vi "HXG2_Timing Module Pump.vi"(7 "Timer Command":T1=enum."Start", 8 "error in (no error)":errorcluster) -> (0 "error out":errorcluster, 1 "Elapsed Time":dbl, 2 "Done?":bool)   [LabVIEW 2012]
doc: "This VI is a functional global variable that keeps track the amount of time elapsed since a Start command was sent to the VI."
uses:
  HXG2_BlowerPumpl.ctl
panel:
  # "Input"
  # "Output"
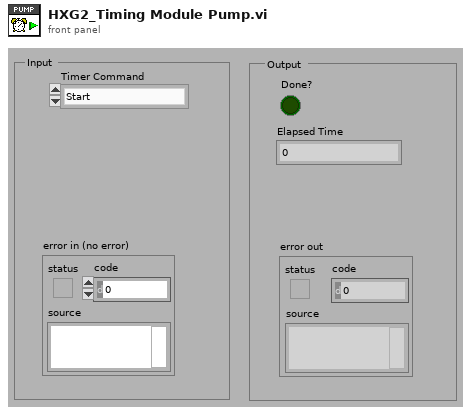
[diagram p1: front panel]
types:
  T1 = typedef "HXG2_BlowerPumpl.ctl" = enum16{"Stop", "Start", "Check Time"}
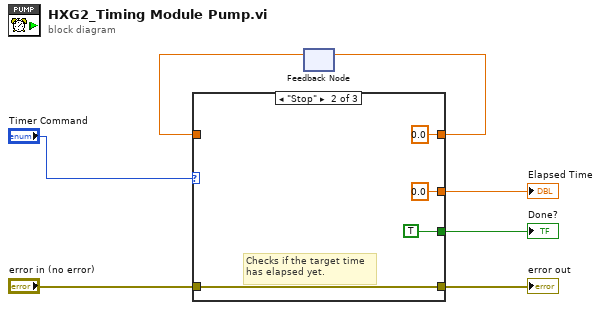
[diagram p0: block diagram]
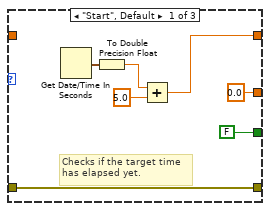
[diagram p2: hidden frame]
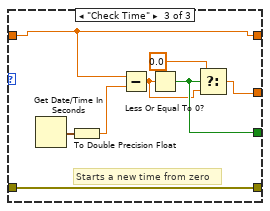
[diagram p3: hidden frame]
diagram:
  n1 = feedback #1() -> (w3:dbl)  [unwired: 1 in]
  n2 = case shown="\"Stop\"" "Timer Command" {
    tunnel: [w10 0.0 w19] -> w4
    tunnel: w3 -> [_ _ w19]
    tunnel: [0.0 ("t") 0.0 ("t") w23] -> w7
    tunnel: [FALSE TRUE w22] -> w6
    tunnel: "error in (no error)" -> [w12 w18 w26]
    tunnel: [w12 w18 w26] -> w1
    frame "Start", Default {
      # "Checks if the target time\nhas elapsed yet."
      n3 = Get Date/Time In Seconds() -> (seconds since 1Jan1904=w14:timestamp)
      n4 = To Double Precision Float(number=w14) -> (double precision float=w13:dbl)
      n5 = Add(x=w13, y=5.0) -> (x+y=w10:dbl)
    }
    frame "Stop" {
      # "Checks if the target time\nhas elapsed yet."
    }
    frame "Check Time" {
      # "Starts a new time from zero"
      n6 = Get Date/Time In Seconds() -> (seconds since 1Jan1904=w25:timestamp)
      n7 = To Double Precision Float(number=w25) -> (double precision float=w20:dbl)
      n8 = Subtract(x=w19, y=w20) -> (x-y=w21:dbl)
      n9 = Less Or Equal To 0?(x=w21) -> (x <= 0?=w22:bool)
      n10 = Select(t=0.0, s=w22, f=w21) -> (s? t:f=w23:dbl)
    }
  }
  "error out" <- w1
  "Elapsed Time" <- w7
  "Done?" <- w6
  n11 = feedback-in #1(w4) -> ()
